vi "Error Handler.vi"(8 "error in (no error)":errorcluster, 9 "Function Name":string, 10 "LINX error code":i32, 11 "LINX Base in":refnum<class "LINX Base.lvclass">) -> (0 "error out":errorcluster, 3 "LINX Base out":refnum<class "LINX Base.lvclass">)   [LabVIEW 2020, in "LINX Base.lvclass"]
uses:
  LINX Base.lvclass
  Typedef/Error Type.ctl
  LINX Base.lvclass/LINX Base.ctl
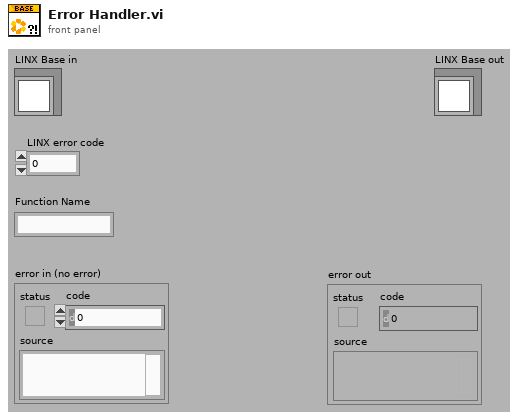
[diagram p1: front panel]
types:
  T1 = typedef "LINX Base.lvclass/Error Type.ctl" = enum16{"Unknown", "Timeout", "Corrupt Return Packet", "Unable To Connect", "Command Not Supported", "Channel DNE", "Invalid COM Config", "Firmware Version Mismatch", "myRIO Support", "CMD Specific Error", "Local IO Not Supported"}
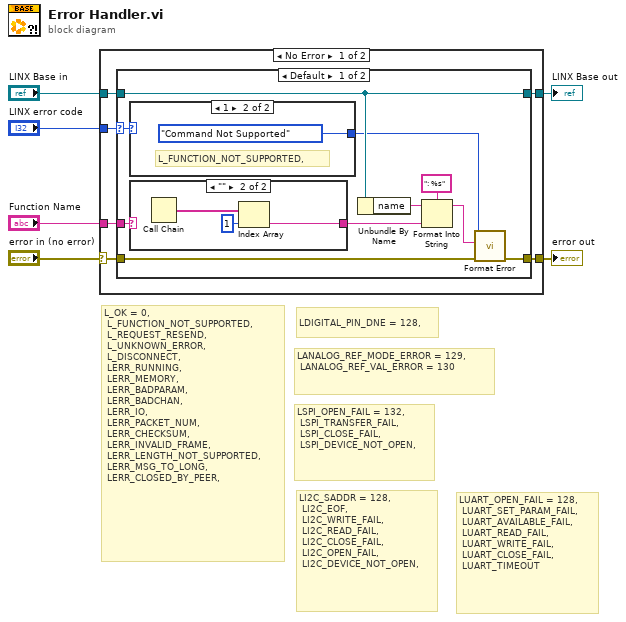
[diagram p0: block diagram]
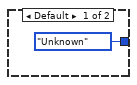
[diagram p3: hidden frame]
diagram:
  # "LUART_OPEN_FAIL = 128,\n\tLUART_SET_PARAM_FAIL,\n\tLUART_AVAILABLE_FAIL,\n\tLUART_READ_FAIL,\n\tLUART_WRITE_FAIL,\n\tLUART_CLOSE_FAIL,\n\tLUART_TIMEOUT"
  # "LI2C_SADDR = 128,\n\tLI2C_EOF,\n\tLI2C_WRITE_FAIL,\n\tLI2C_READ_FAIL,\n\tLI2C_CLOSE_FAIL,\n\tLI2C_OPEN_FAIL,\n\tLI2C_DEVICE_NOT_OPEN,"
  # "LSPI_OPEN_FAIL = 132,\n\tLSPI_TRANSFER_FAIL,\n\tLSPI_CLOSE_FAIL,\n\tLSPI_DEVICE_NOT_OPEN,"
  # "LDIGITAL_PIN_DNE = 128,"
  # "LANALOG_REF_MODE_ERROR = 129,\n\tLANALOG_REF_VAL_ERROR = 130"
  # "L_OK = 0,\n\tL_FUNCTION_NOT_SUPPORTED,\n\tL_REQUEST_RESEND,\n\tL_UNKNOWN_ERROR,\n\tL_DISCONNECT,\n\tLERR_RUNNING,\n\tLERR_MEMORY,\n\tLERR_BADPARAM,\n\tLERR_BADCHAN,\n\tLERR_IO,\n\tLERR_PACKET_NUM,\n\tLERR_CHECKSUM,\n\tLERR_INVALID_FRAME,\n\tLERR_LENGTH_NOT_SUPPORTED,\n\tLERR_MSG_TO_LONG,\n\tLERR_CLOSED_BY_PEER,"
  n1 = case shown="No Error" "error in (no error)" {
    selector: "error in (no error)" -> [w9 w31]
    tunnel: "LINX error code" -> [w11 _]
    tunnel: "LINX Base in" -> [w12 w32]
    tunnel: [w10 w32] -> w2
    tunnel: [w8 w31] -> w3
    tunnel: "Function Name" -> [w7 _]
    frame No Error {
      n2 = case shown="Default" w11 {
        selector: w11 -> [w19 _]
        tunnel: w12 -> [w22 w30]
        tunnel: [w22 w30] -> w10
        tunnel: [w15 w29] -> w8
        tunnel: w9 -> [w18 w29]
        tunnel: w7 -> [w14 _]
        frame Default {
          n3 = case shown="1" w19 {
            tunnel: [Error_Type."Unknown" ("Error Type") Error_Type."Command Not Supported" ("Error Type")] -> w16
            frame Default {
            }
            frame 1 {
              # "L_FUNCTION_NOT_SUPPORTED,"
            }
          }
          n4 = case shown="\"\"" w14 {
            selector: w14 -> [w23 _]
            tunnel: [w23 w24] -> w13
            frame Default {
            }
            frame "" {
              n5 = Call Chain() -> (call chain=w26:string[])
              n6 = Index Array(array=w26, index=1) -> (element=w24:string)
            }
          }
          n7 = Unbundle By Name(w22) -> ("name"=w20:string)
          n8 = Format Into String(format string=": %s", initial string=w20, w13) -> (resulting string=w17:string)  [unwired: 1 in, 1 out]
          n9 = call "Format Error.vi"("error in (no error)"=w18, "Message"=w17, "Error Type"=w16) -> ("error out"=w15:errorcluster)  [unwired: 8 out]
        }
        frame 0 {
          # "L_OK"
        }
      }
    }
    frame Error {
    }
  }
  "error out" <- w3
  "LINX Base out" <- w2
